vi "VISJS_SendDataToWebBrowser.vi"   [LabVIEW 2020, in "VISJS Viewer.lvlib"]
uses:
  b3c0b3e7-f247-474e-8f48-bbd2c77c245b.vi
  VISJS Viewer.lvlib
types:
  T1 = enum16{"Standard", "Buffered", "CRLF", "Immediate"}
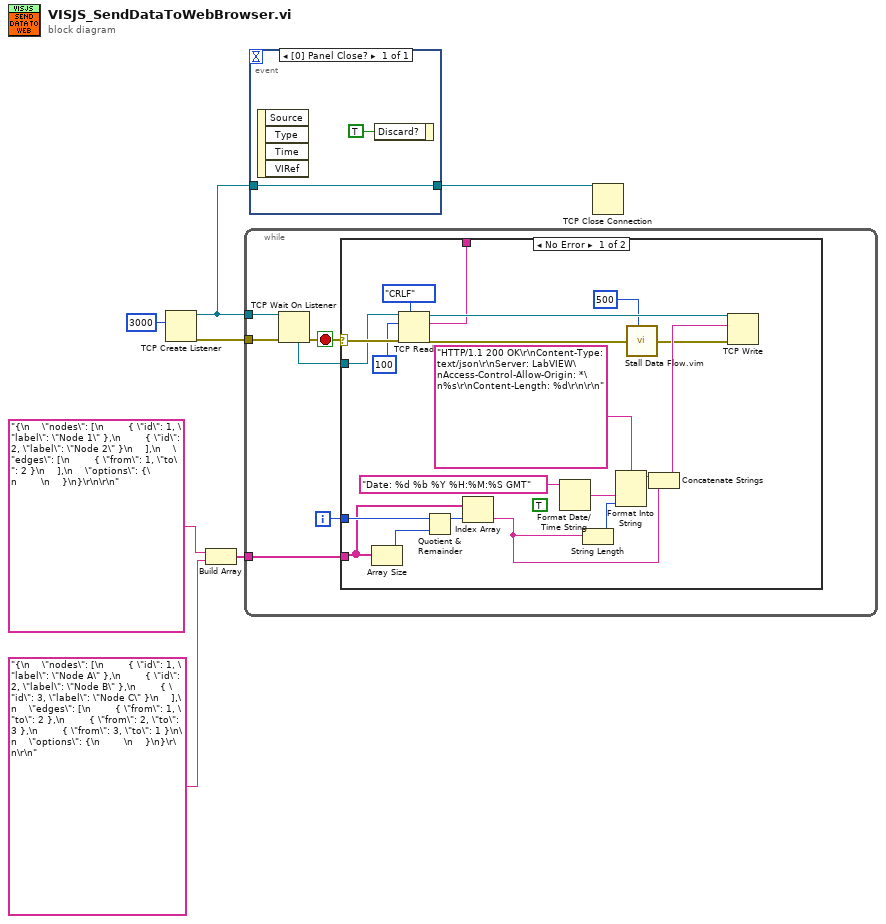
[diagram p0: block diagram]
diagram:
  n1 = TCP Create Listener(10:u16 3000 ("port")) -> (0:w6:errorcluster, 3:w5:refnum<k5>)  [unwired: 4 in, 1 out]
  n2 = Build Array("{\n    \"nodes\": [\n        { \"id\": 1, \"label\": \"Node 1\" },\n        { \"id\": 2, \"label\": \"Node 2\" }\n    ],\n    \"edges\": [\n        { \"from\": 1, \"to\": 2 }\n    ],\n    \"options\": {\n        \n    }\n}\r\n\r\n", "{\n    \"nodes\": [\n        { \"id\": 1, \"label\": \"Node A\" },\n        { \"id\": 2, \"label\": \"Node B\" },\n        { \"id\": 3, \"label\": \"Node C\" }\n    ],\n    \"edges\": [\n        { \"from\": 1, \"to\": 2 },\n        { \"from\": 2, \"to\": 3 },\n        { \"from\": 3, \"to\": 1 }\n\n    \"options\": {\n        \n    }\n}\r\n\r\n") -> (w1:string[])
  n3 = while {
    tunnel: w6 -> [w13]
    tunnel: w5 -> [w12]
    tunnel: w1 -> [w9]
    i -> [w8]
    stop <- w11 stop-if-true
    n4 = TCP Wait On Listener(8:w13, 11:w12) -> (0:w11:errorcluster, 4:w10:refnum<k5>)  [unwired: 2 in, 3 out]
    n5 = case shown="No Error" w11 {
      selector: w11 -> [w33 _]
      tunnel: w10 -> [w31 _]
      tunnel: [w27 _] -> _
      tunnel: w9 -> [w18 _]
      tunnel: w8 -> [w20 _]
      frame No Error {
        (unwired) TRUE ("UTC format")
        n6 = Array Size(array=w18) -> (size(s)=w19:i32)
        n7 = TCP Read(connection ID=w31, bytes to read=100, error in (no error)=w33, 7:T1."CRLF" ("mode (standard)")) -> (connection ID out=w28:refnum<k5>, data out=w27:string, error out=w22:errorcluster)  [unwired: 1 in]
        n8 = Quotient & Remainder(x=w20, y=w19) -> (x-y*floor(x/y)=w17:i32)  [unwired: 1 out]
        n9 = Index Array(array=w18, index=w17) -> (element=w16:string)
        n10 = Format Date/Time String(time format string (%c)="Date: %d %b %Y %H:%M:%S GMT") -> (date/time string=w24:string)  [unwired: 2 in]
        n11 = String Length(string=w16) -> (length=w23:i32)
        n12 = Format Into String(format string="HTTP/1.1 200 OK\r\nContent-Type: text/json\r\nServer: LabVIEW\nAccess-Control-Allow-Origin: *\n%s\r\nContent-Length: %d\r\n\r\n", w24, w23) -> (resulting string=w26:string)  [unwired: 2 in, 1 out]
        n13 = call "Stall Data Flow.vim"("value in"=w22, "milliseconds to wait"=u32 500) -> ("value out"=w15:errorcluster)  [unwired: 1 out]
        n14 = Concatenate Strings(w26, w16) -> (w21:string)
        n15 = TCP Write(connection ID=w28, data in=w21, error in (no error)=w15) -> ()  [unwired: 1 in, 3 out]
      }
      frame Error {
      }
    }
  }
  n16 = event shown="[0] Panel Close?" {
    selector: _ -> [_]
    dyn-events: _ -> [_]
    timeout: _ -> [_]
    tunnel: w5 -> [w34]
    tunnel: [w34] -> w4
    event Panel Close? {
      n17 = event-data() -> ()  [unwired: 1 in, 4 out]
      n18 = event-data("Discard?"=TRUE) -> ()  [unwired: 1 in, 1 out]
    }
  }
  n19 = TCP Close Connection(connection ID=w4) -> ()  [unwired: 2 in, 2 out]
